vi "Read Multi-D.vi"(8 "Error In":errorcluster, 9 "Length (U16)":u16, 10 "Start Position (U32)":u32, 11 "connection ID":refnum<k5>) -> (0 "Error Out":errorcluster, 2 "D Data out":i16[](array[numeric]), 3 "connection ID out":refnum<k5>)   [LabVIEW 2019, in "FX5U SLMP Binary.lvlib"]
uses:
  FX5U SLMP Binary.lvlib
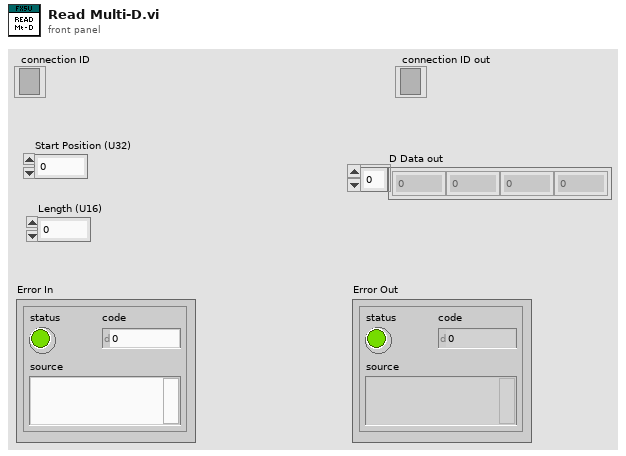
[diagram p1: front panel]
types:
  T1 = enum16{"big-endian, network order", "native, host order", "little-endian"}
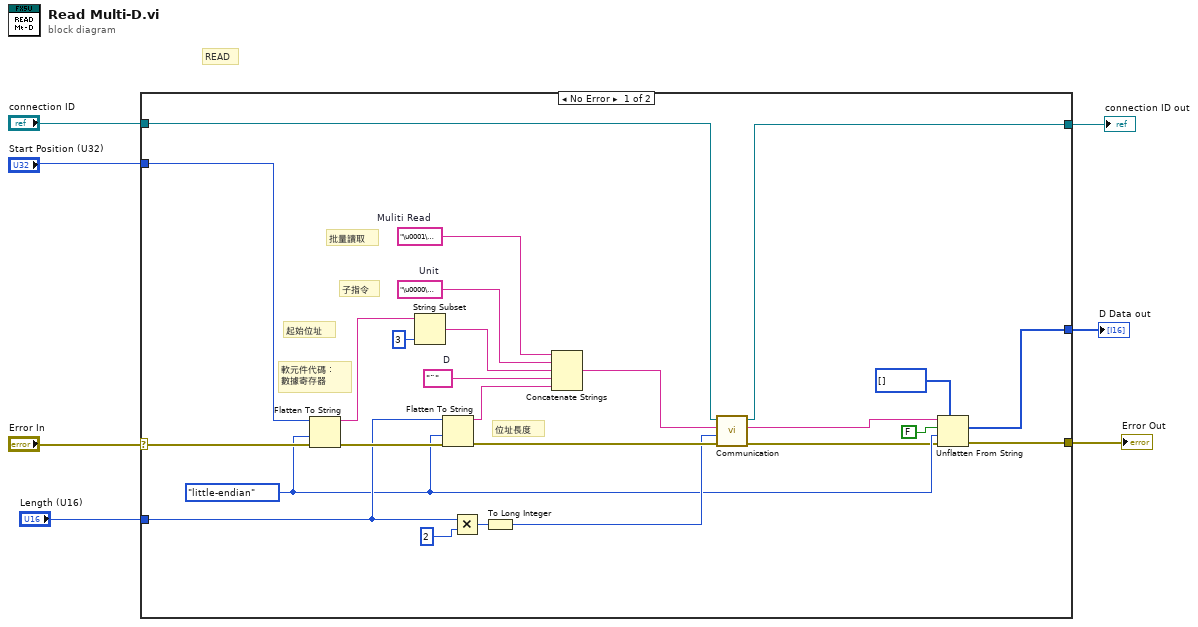
[diagram p0: block diagram]
diagram:
  # "READ"
  n1 = case shown="No Error" "Error In" {
    selector: "Error In" -> [w23 w34]
    tunnel: [w9 w34] -> w7
    tunnel: [w8 _] -> w1
    tunnel: "Start Position (U32)" -> [w24 _]
    tunnel: "Length (U16)" -> [w16 _]
    tunnel: "connection ID" -> [w20 w33]
    tunnel: [w19 w33] -> w2
    frame No Error {
      w12 = T1."little-endian" ("byte order (0:big-endian, network order)")
      w27 = "¨"  # D
      w31 = "\u0000\u0000"  # Unit
      w32 = "\u0001\u0004"  # Muliti Read
      # "位址長度"
      # "軟元件代碼 : \n數據寄存器"
      # "起始位址"
      # "子指令"
      # "批量讀取"
      n2 = Flatten To String(anything=w24, byte order (0:big-endian, network order)=w12, error in (no error)=w23) -> (data string=w29:string, error out=w26:errorcluster)  [unwired: 1 in, 1 out]
      n3 = String Subset(string=w29, length (rest)=3 ("length (rest)")) -> (substring=w30:string)  [unwired: 1 in]
      n4 = Flatten To String(anything=w16, byte order (0:big-endian, network order)=w12, error in (no error)=w26) -> (data string=w25:string, error out=w22:errorcluster)  [unwired: 1 in, 1 out]
      n5 = Multiply(x=w16, y=u16 2) -> (x*y=w15:u16)
      n6 = To Long Integer(number=w15) -> (32bit integer=w18:i32)
      n7 = Concatenate Strings(w32, w31, w30, w27, w25) -> (w21:string)
      n8 = call "Communication.vi"("Error In"=w22, "Bytes to Read(I32)"=w18, "Command"=w21, "connection ID"=w20) -> ("Error Out"=w11:errorcluster, "Data out"=w10:string, "connection ID out"=w19:refnum<k5>)  [unwired: 5 in]
      n9 = Unflatten From String(type=i16[] [], binary string=w10, data includes array or string size? (T)=FALSE, byte order (0:big-endian, network order)=w12, error in (no error)=w11) -> (value=w8:i16[], error out=w9:errorcluster)  [unwired: 1 out]
    }
    frame Error {
    }
  }
  "Error Out" <- w7
  "connection ID out" <- w2
  "D Data out" <- w1
